vi "test4.vi"   [LabVIEW 2020]
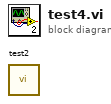
[diagram p0: block diagram]
diagram:
  n1 = call "test2.vi"() -> ()  [unwired: 12 in]
